vi "prepareCmdStatus.vi"(8 "error in (no error)":errorcluster, 9 "cmdStatus":string(combo)="ack", 10 "tcpPacket":string, 11 "tcpServerCmd in":refnum<class "TcpServerCmd.lvclass">) -> (0 "error out":errorcluster, 3 "tcpServerCmd out":refnum<class "TcpServerCmd.lvclass">)   [LabVIEW 2018, in "TcpServerCmd.lvclass"]
doc: "Prepare cmd Status."
uses:
  TcpServerCmd.lvclass
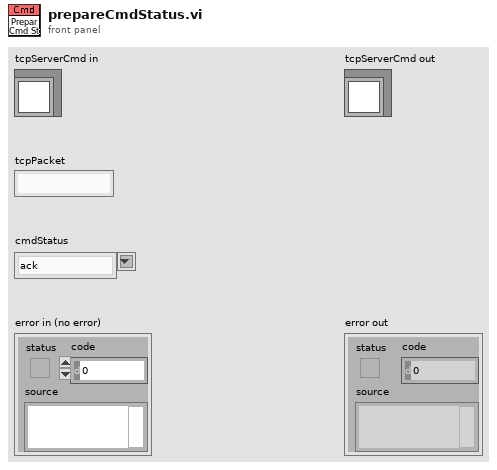
[diagram p1: front panel]
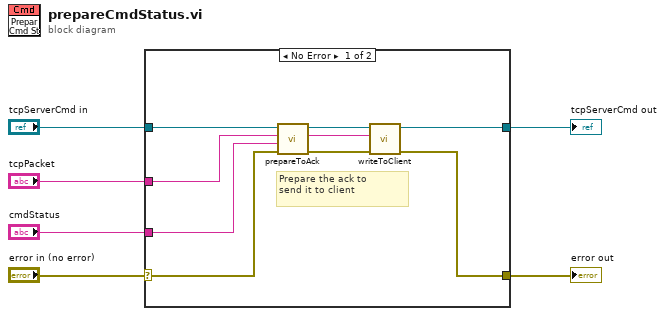
[diagram p0: block diagram]
diagram:
  n1 = case shown="No Error" "error in (no error)" {
    selector: "error in (no error)" -> [w11 w17]
    tunnel: [w14 w17] -> w5
    tunnel: [w15 w16] -> w3
    tunnel: "tcpServerCmd in" -> [w13 w16]
    tunnel: "cmdStatus" -> [w9 _]
    tunnel: "tcpPacket" -> [w8 _]
    frame No Error {
      # "Prepare the ack to\nsend it to client"
      n2 = call "prepareToAck.vi"("error in (no error)"=w11, "cmdStatus"=w9, "cmd"=w8, "tcpServerCmd in"=w13) -> ("error out"=w10:errorcluster, "JSON string"=w7:string, "tcpServerCmd out"=w12:refnum<class "TcpServerCmd.lvclass">)  [unwired: 5 in]
      n3 = call "writeToClient.vi"("error in (no error)"=w10, "packet"=w7, "tcpServerCmd in"=w12) -> ("error out"=w14:errorcluster, "tcpServerCmd out"=w15:refnum<class "TcpServerCmd.lvclass">)  [unwired: 7 in]
    }
    frame Error {
    }
  }
  "error out" <- w5
  "tcpServerCmd out" <- w3
